vi "Ignore Folders.vi"(3 "File":path, 4 "Ignore Folders":path[](array[path])) -> (0 "index of element":i32)   [LabVIEW 2015]
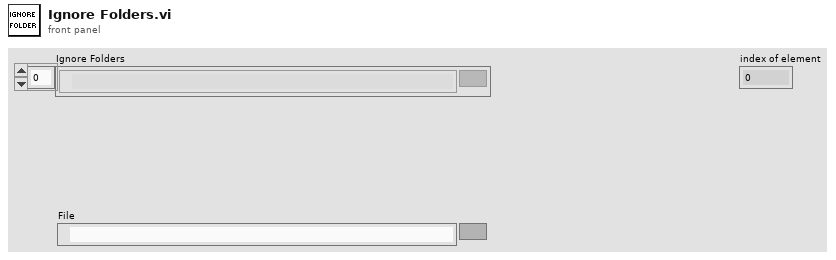
[diagram p1: front panel]
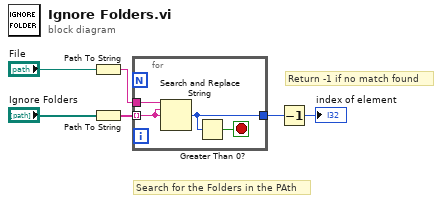
[diagram p0: block diagram]
diagram:
  # "Return -1 if no match found"
  # "Search for the Folders in the PAth"
  n1 = Path To String(path="File") -> (string=w6:string)
  n2 = Path To String(path="Ignore Folders") -> (string=w5:string[])
  n3 = for {
    tunnel: w6 -> [w10]
    tunnel: w5 -> [w9] mode=indexing
    tunnel: [w7] -> w4
    stop <- w8 stop-if-true
    n4 = Search and Replace String(input string=w10, search string=w9, replace string=w9) -> (number of replacements=w7:i32)  [unwired: 5 in, 3 out]
    n5 = Greater Than 0?(x=w7) -> (x > 0?=w8:bool)
  }
  n6 = Decrement(x=w4) -> (x-1=→"index of element":i32)
